vi "Errors.vi"(8 "error in (no error)":errorcluster, 11 "Node Ptr":T2 format="%.0x") -> (0 "error out":errorcluster)   [LabVIEW 2015, in "Development Tools Examples System Explorer.lvlib"]
uses:
  Development Tools Examples System Explorer.lvlib
  <vilib>/NI Veristand/Custom Device API/Custom Device Item Ref.ctl
  <vilib>/NI/VeriStand Error API/VeriStand Error.ctl
  <vilib>/NI Veristand/Custom Device API/Custom Device API.lvlib
  <vilib>/NI/VeriStand Error API/VeriStand Error API.lvlib
panel:
  in  "Clear All Errors":bool
  in  "Clear Error":bool
  in  "Errors":i32(listbox)
  in  "Clear Manual Error":bool
  in  "Throw Error":bool
  in  "VeriStand Error In":T1
  in  "Key":string
  out "VeriStand Errors":T1[](array[typedef])
  in  "Header":cluster{"Section Name":string}={"Section Name"="Custom Device Item Settings"}
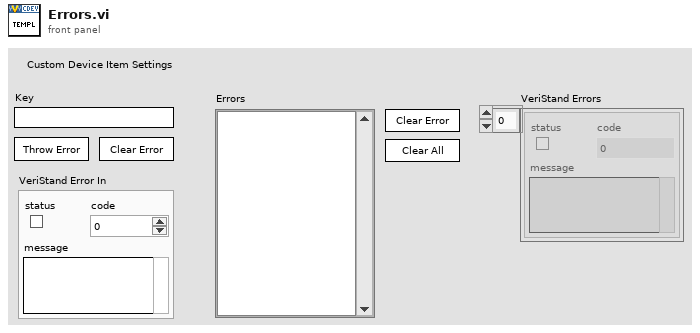
[diagram p1: front panel]
types:
  T1 = typedef "VeriStand Error API.lvlib/VeriStand Error.ctl" = cluster{"status":bool, "code":i32, "message":string}
  T2 = typedef "Custom Device API.lvlib/Custom Device Item Ref.ctl" = u64
  T3 = typedef "Custom Device API.lvlib/Custom Device Commands.ctl" = enum16{"Default", "Item renamed", "Shutdown", "Dynamic button pressed"}
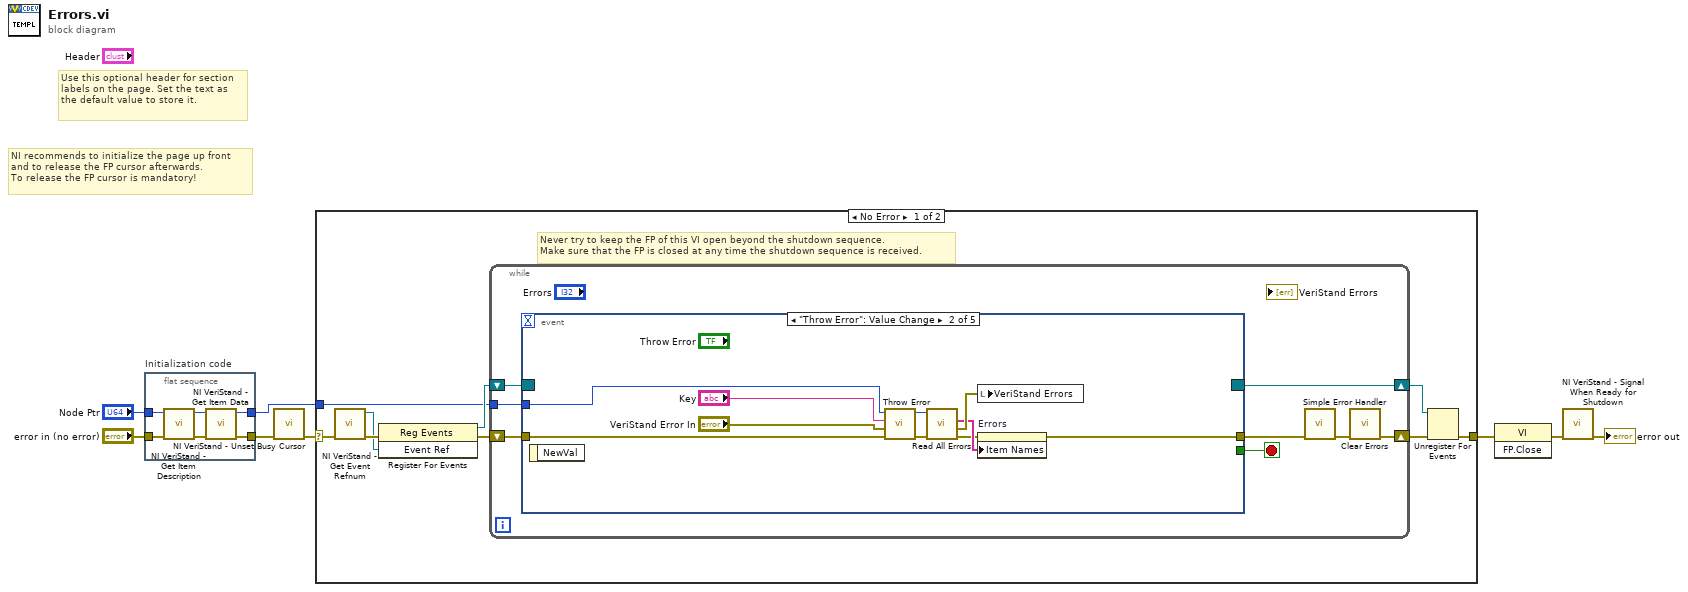
[diagram p0: block diagram]
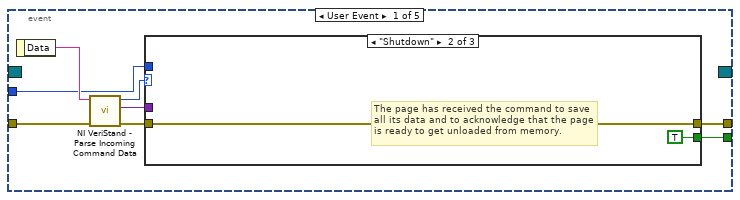
[diagram p2: hidden frame]
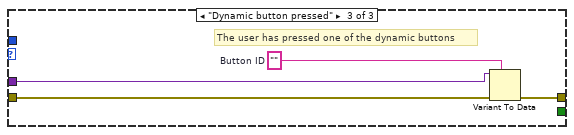
[diagram p4: hidden frame]
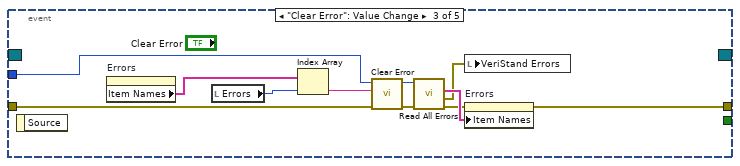
[diagram p5: hidden frame]
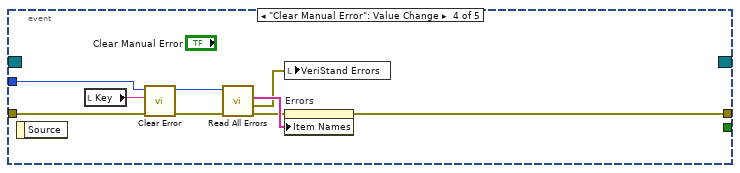
[diagram p6: hidden frame]
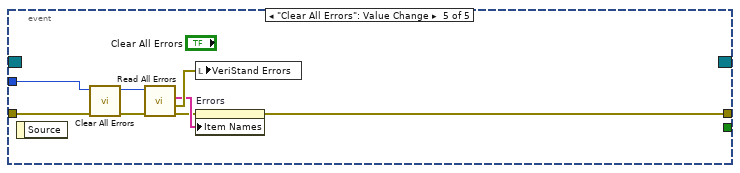
[diagram p7: hidden frame]
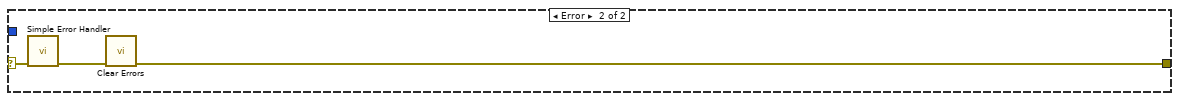
[diagram p8: hidden frame]
diagram:
  # "Use this optional header for section labels on the page. Set the text as the default value to store it."
  # "NI recommends to initialize the page up front\nand to release the FP cursor afterwards.\nTo release the FP cursor is mandatory!"
  n1 = flat-sequence "Initialization code" {
    tunnel: "error in (no error)" -> [w12]
    tunnel: "Node Ptr" -> [w11]
    tunnel: [w9] -> w6
    tunnel: [w14] -> w5
    frame #0 {
      n2 = call <vilib>:"NI VeriStand - Get Item Description.vi"("error in (no error)"=w12, "Item Ref in"=w11) -> ("error out"=w10:errorcluster, "Item Ref out"=w13:T2)  [unwired: 8 out]
      n3 = call <vilib>:"NI VeriStand - Get Item Data.vi"("error in (no error)"=w10, "Item Ref in"=w13) -> ("error out"=w9:errorcluster, "Item Ref out"=w14:T2)  [unwired: 8 out]
    }
  }
  n4 = call <vilib>:"NI VeriStand - Unset Busy Cursor.vi"("error in (no error)"=w6) -> ("error out"=w4:errorcluster)  [unwired: 10 out]
  n5 = case shown="No Error" w4 {
    selector: w4 -> [w15 w87]
    tunnel: [w20 w85] -> w1
    tunnel: w5 -> [w16 _]
    frame No Error {
      # "Never try to keep the FP of this VI open beyond the shutdown sequence.\nMake sure that the FP is closed at any time the shutdown sequence is received."
      n6 = call <vilib>:"NI VeriStand - Get Event Refnum.vi"("error in (no error)"=w15) -> ("error out"=w23:errorcluster, "Event Ref"=w19:refnum<user-event>)  [unwired: 9 out]
      n7 = register-events(error in=w23, w19) -> (reference out=w17:refnum<event-registration>, error out=w18:errorcluster)  [unwired: 1 in]
      n8 = while {
        tunnel: w16 -> [w27]
        shift-right: [w24] -> w21
        shift-left: w18 -> [w30]
        shift-right: [w31] -> w22
        shift-left: w17 -> [w29]
        stop <- w28 stop-if-true
        n9 = event shown="[1] \"Throw Error\": Value Change" {
          selector: w29 -> [_ _ _ _ _]
          dyn-events: [_ _ _ _ _] -> w31
          timeout: _ -> [_ _ _ _ _]
          tunnel: w30 -> [w39 w56 w65 w74 w82]
          tunnel: [w35 _ _ _ _] -> w28
          tunnel: [w34 w49 w58 w70 w77] -> w26
          tunnel: w27 -> [w33 w47 w66 w75 w81]
          event User Event {
            n10 = event-data() -> ("Data"=w38:string)  [unwired: 1 out]
            n11 = call <vilib>:"NI VeriStand - Parse Incoming Command Data.vi"("error in (no error)"=w39, "Incoming data"=w38) -> ("error out"=w37:errorcluster, "Outgoing data"=w32:variant, "Action"=w36:T3)  [unwired: 7 out]
            n12 = case shown="\"Shutdown\"" w36 {
              tunnel: w37 -> [w40 w41 w46]
              tunnel: [_ TRUE _] -> w35
              tunnel: [w40 w41 w43] -> w34
              tunnel: w33 -> [_ _ _]
              tunnel: w32 -> [_ _ w45]
              frame "Default", Default {
              }
              frame "Shutdown" {
                # "The page has received the command to save all its data and to acknowledge that the page is ready to get unloaded from memory."
              }
              frame "Dynamic button pressed" {
                w44 = ""  # Button ID
                # "The user has pressed one of the dynamic buttons"
                n13 = Variant To Data(error in=w46, type=w44, Variant=w45) -> (error out=w43:errorcluster)  [unwired: 1 out]
              }
            }
          }
          event "Throw Error": Value Change {
            n14 = event-data() -> ()  [unwired: 2 out]
            n15 = call <vilib>:"Throw Error.vi"("error in"=w56, "VeriStand Error In"="VeriStand Error In", "Key"="Key", "Item Ref in"=w47) -> ("error out"=w53:errorcluster, "Item Ref out"=w54:T2)  [unwired: 6 in]
            n16 = call <vilib>:"Read All Errors.vi"("error in (no error)"=w53, "Item Ref in"=w54) -> ("error out"=w50:errorcluster, "VeriStand Errors"=w52:T1[], "Keys"=w51:string[])  [unwired: 6 in, 1 out]
            n17 = local write "VeriStand Errors"(w52) -> ()
            n18 = property on="Errors" class="LstBox (strict)"(error in=w50, "Item Names"=w51) -> (error out=w49:errorcluster)  [unwired: 1 in, 1 out]
          }
          event "Clear Error": Value Change {
            n19 = event-data() -> ()  [unwired: 2 out]
            n20 = property on="Errors" class="LstBox (strict)"() -> ("Item Names"=w62:string[])  [unwired: 2 in, 2 out]
            n21 = local read "Errors"() -> (w61:i32)
            n22 = Index Array(array=w62, index=w61) -> (element=w60:string)
            n23 = call <vilib>:"Clear Error.vi"("error in (no error)"=w65, "Key"=w60, "Item Ref in"=w66) -> ("error out"=w64:errorcluster, "Item Ref out"=w67:T2)  [unwired: 7 in]
            n24 = call <vilib>:"Read All Errors.vi"("error in (no error)"=w64, "Item Ref in"=w67) -> ("error out"=w59:errorcluster, "VeriStand Errors"=w57:T1[], "Keys"=w63:string[])  [unwired: 6 in, 1 out]
            n25 = local write "VeriStand Errors"(w57) -> ()
            n26 = property on="Errors" class="LstBox (strict)"(error in=w59, "Item Names"=w63) -> (error out=w58:errorcluster)  [unwired: 1 in, 1 out]
          }
          event "Clear Manual Error": Value Change {
            n27 = event-data() -> ()  [unwired: 2 out]
            n28 = local read "Key"() -> (w68:string)
            n29 = call <vilib>:"Clear Error.vi"("error in (no error)"=w74, "Key"=w68, "Item Ref in"=w75) -> ("error out"=w73:errorcluster, "Item Ref out"=w76:T2)  [unwired: 7 in]
            n30 = call <vilib>:"Read All Errors.vi"("error in (no error)"=w73, "Item Ref in"=w76) -> ("error out"=w71:errorcluster, "VeriStand Errors"=w69:T1[], "Keys"=w72:string[])  [unwired: 6 in, 1 out]
            n31 = local write "VeriStand Errors"(w69) -> ()
            n32 = property on="Errors" class="LstBox (strict)"(error in=w71, "Item Names"=w72) -> (error out=w70:errorcluster)  [unwired: 1 in, 1 out]
          }
          event "Clear All Errors": Value Change {
            n33 = event-data() -> ()  [unwired: 2 out]
            n34 = call <vilib>:"Clear All Errors.vi"("error in (no error)"=w82, "Item Ref in"=w81) -> ("error out"=w83:errorcluster, "Item Ref out"=w84:T2)  [unwired: 8 in]
            n35 = call <vilib>:"Read All Errors.vi"("error in (no error)"=w83, "Item Ref in"=w84) -> ("error out"=w78:errorcluster, "VeriStand Errors"=w80:T1[], "Keys"=w79:string[])  [unwired: 6 in, 1 out]
            n36 = local write "VeriStand Errors"(w80) -> ()
            n37 = property on="Errors" class="LstBox (strict)"(error in=w78, "Item Names"=w79) -> (error out=w77:errorcluster)  [unwired: 1 in, 1 out]
          }
        }
        n38 = call <vilib>:"Simple Error Handler.vi"("error in (no error)"=w26) -> ("error out"=w25:errorcluster)  [unwired: 1 in, 7 out]
        n39 = call <vilib>:"Clear Errors.vi"("error in (no error)"=w25) -> ("error out"=w24:errorcluster)  [unwired: 1 in, 5 out]
      }
      n40 = Unregister For Events(event registration refnum=w22, error in=w21) -> (error out=w20:errorcluster)
    }
    frame Error {
      n41 = call <vilib>:"Simple Error Handler.vi"("error in (no error)"=w87) -> ("error out"=w86:errorcluster)  [unwired: 1 in, 7 out]
      n42 = call <vilib>:"Clear Errors.vi"("error in (no error)"=w86) -> ("error out"=w85:errorcluster)  [unwired: 1 in, 5 out]
    }
  }
  n43 = invoke class="VI" method="FP.Close"(error in=w1) -> (error out=w8:errorcluster)  [unwired: 2 in, 2 out]
  n44 = call <vilib>:"NI VeriStand - Signal When Ready for Shutdown.vi"("error in (no error)"=w8) -> ("error out"=→"error out":errorcluster)  [unwired: 10 out]
